vi "onCreate.vi"(8 "error in (no error)":errorcluster, 11 "Server in":refnum<class "Server.lvclass">) -> (0 "error out":errorcluster, 3 "Server out":refnum<class "Server.lvclass">)   [LabVIEW 2013, in "MQTT Server.lvlib" / "Server.lvclass"]
uses:
  Server.lvclass
  SessionRef -- cluster.ctl
  <vilib>/LabVIEW Open Source Project/MQTT Connection/MQTT_Base/Base Class/Response -- cluster.ctl
  <vilib>/LabVIEW Open Source Project/MQTT Control Packets/Control Packets/ControlPacket/ControlPacket.lvclass
  Subscription/_Subscription.lvclass
  Private Events -- cluster.ctl
  <vilib>/LabVIEW Open Source Project/MQTT Control Packets/Control Packets/PUBLISH/PUBLISH.lvclass
  <vilib>/LabVIEW Open Source Project/MQTT Control Packets/Control Packets/Ack/Ack.lvclass
  <vilib>/LabVIEW Open Source Project/MQTT Connection/MQTT_Base/Base Class/MQTT_Base.lvclass
  Server.lvclass/Server.ctl
  StoredSessions/StoredSessions.lvclass
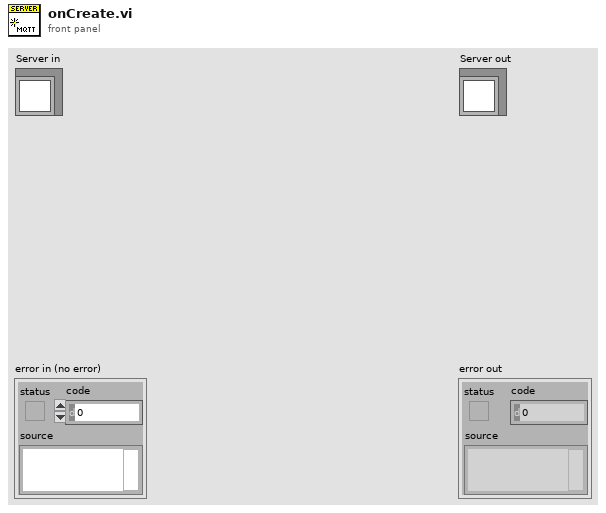
[diagram p1: front panel]
types:
  T1 = typedef "MQTT Server.lvlib/Server.lvclass/Private Events -- cluster.ctl" = cluster{"Inbound Packet":refnum<user-event>, "Inbound Ack":refnum<user-event>}
  T2 = typedef "MQTT Server.lvlib/Server.lvclass/SessionRef -- cluster.ctl" = cluster{"ClientID":string, "SessionMailbox":refnum<queue>}
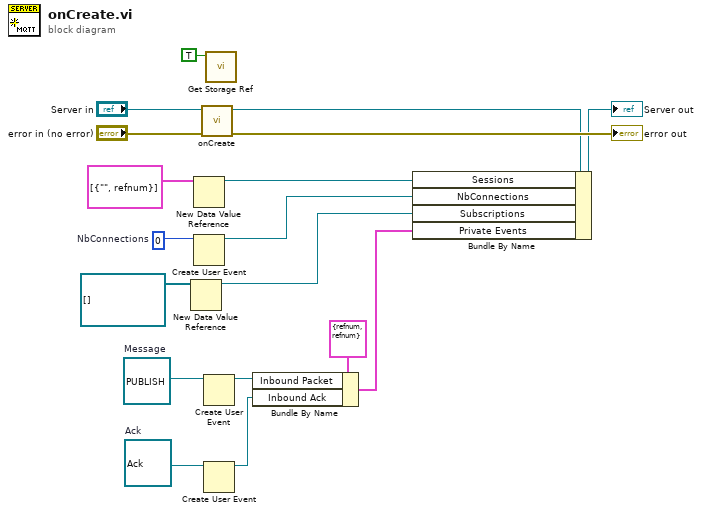
[diagram p0: block diagram]
diagram:
  w3 = refnum<class "Ack.lvclass"> refnum  # Ack
  w4 = refnum<class "PUBLISH.lvclass"> refnum  # Message
  w12 = u32 0  # NbConnections
  n1 = New Data Value Reference(data value=refnum<class "_Subscription.lvclass">[] []) -> (data value reference=w7:refnum<data-value>)  [unwired: 1 in, 1 out]
  n2 = New Data Value Reference(data value=T2[] [{"ClientID"="", "SessionMailbox"=refnum}]) -> (data value reference=w14:refnum<data-value>)  [unwired: 1 in, 1 out]
  n3 = Create User Event(user event datatype=w12) -> (user event=w11:refnum<user-event>)  [unwired: 1 in, 1 out]
  n4 = call-parent "onCreate.vi"("error in (no error)"="error in (no error)", "MQTT_Base in"="Server in") -> ("error out"=→"error out":errorcluster, "MQTT_Base out"=w13:refnum<class "Server.lvclass">)  [unwired: 8 in]
  n5 = Create User Event(user event datatype=w4) -> (user event=w5:refnum<user-event>)  [unwired: 1 in, 1 out]
  n6 = Create User Event(user event datatype=w3) -> (user event=w2:refnum<user-event>)  [unwired: 1 in, 1 out]
  n7 = call "Get Storage Ref.vi"("Init (F)"=TRUE) -> ()  [unwired: 10 in, 1 out]
  n8 = Bundle By Name(cluster=T1 {"Inbound Packet"=refnum, "Inbound Ack"=refnum} ("Private Events"), "Inbound Packet"=w5, "Inbound Ack"=w2) -> (w1:T1)
  n9 = Bundle By Name(cluster=w13, "Sessions"=w14, "NbConnections"=w11, "Subscriptions"=w7, "Private Events"=w1) -> (→"Server out":refnum<class "Server.lvclass">)
